vi "Enable S-parameter Table.vi"(8 "error in (no error)":errorcluster, 10 "Enable S-parameter Correction (T: Enable)":bool=TRUE, 11 "VISA resource name":refnum<visa-resource-name>) -> (0 "error out":errorcluster, 3 "VISA resource name out":refnum<visa-resource-name>)   [LabVIEW 2014, in "Agilent U2000 Series.lvlib"]
doc: "Enables or disables the S-parameter correction.\nWhen this is enabled, S-parameter values from the selected S-parameter table will be used for correction.\n\nNote: \nThis VI is only applicable for U2040 X-Series."
uses:
  Agilent U2000 Series.lvlib
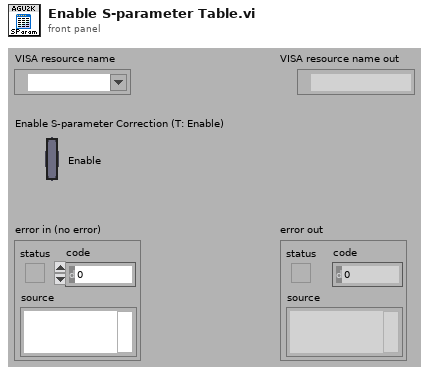
[diagram p1: front panel]
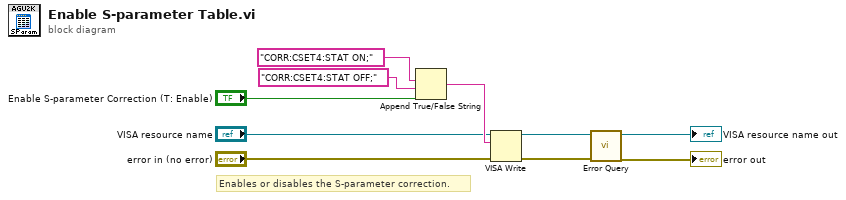
[diagram p0: block diagram]
diagram:
  # "Enables or disables the S-parameter correction."
  n1 = Append True/False String(1:"Enable S-parameter Correction (T: Enable)", 2:"CORR:CSET4:STAT OFF;", 3:"CORR:CSET4:STAT ON;") -> (0:w7:string)  [unwired: 1 in]
  n2 = VISA Write(VISA resource name="VISA resource name", write buffer=w7, error in (no error)="error in (no error)") -> (VISA resource name out=w4:refnum<visa-resource-name>, error out=w3:errorcluster)  [unwired: 1 out]
  n3 = call "Error Query.vi"("error in (no error)"=w3, "VISA resource name"=w4) -> ("error out"=→"error out":errorcluster, "VISA resource name out"=→"VISA resource name out":refnum<visa-resource-name>)  [unwired: 6 in, 2 out]
